vi "Main.vi"() -> ()   [LabVIEW 2016]
uses:
  Composite/Composite Waveform.lvclass
  C:/Users/fflores/Documents/LabVIEW-Open-Projects/Signal Generator OOP/Waveform/Waveform.lvclass
  Sine/Sine.lvclass
  Triangle/Triangle.lvclass
  Waveform/Waveform.lvclass/Waveform.ctl
  Composite/Composite Waveform.lvclass/Composite Waveform.ctl
  Waveform/Waveform.lvclass
panel:
  in  "Refresh Button":bool
  in  "Select Specific Waveform":i32
  in  "Remove Button":bool
  out "Waveform Graph 2":waveform(dbl)(graph)
  in  "Add":bool
  in  "Waveform":enum16{"Sine", "Todas", "Triangle"}(ring)
  in  "stop":bool
  in  "Amplitude":dbl
  in  "Offset":dbl
  in  "Frequency":dbl
  out "Waveform Graph":waveform(dbl)(graph)
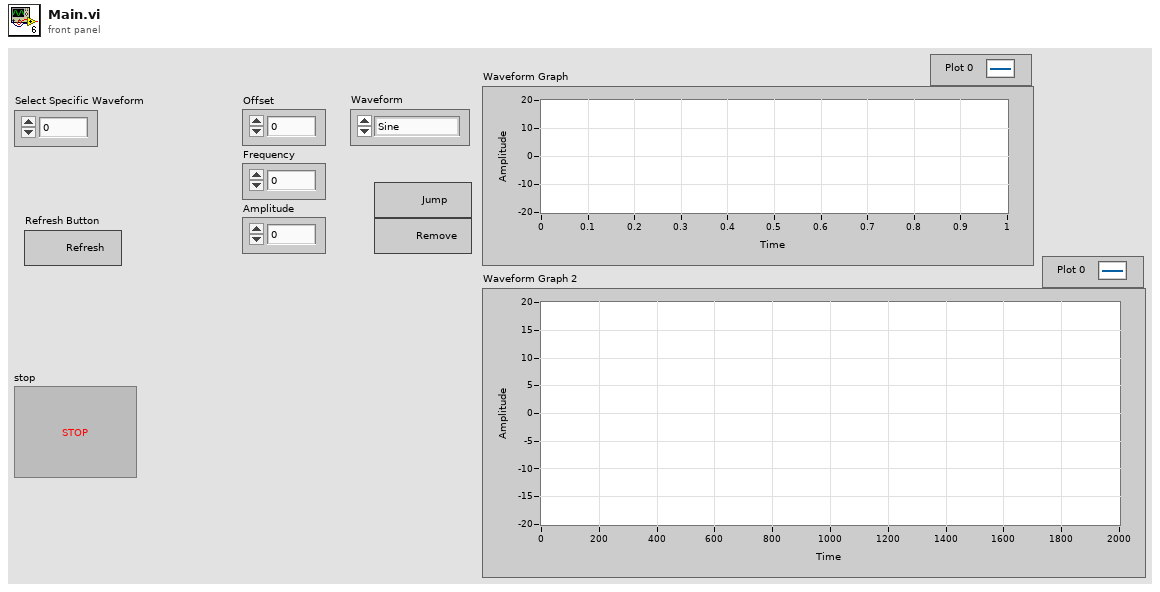
[diagram p1: front panel]
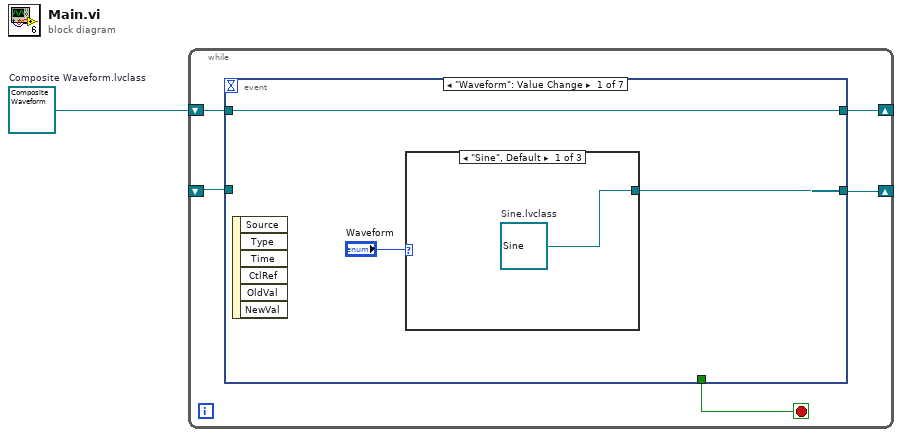
[diagram p0: block diagram]
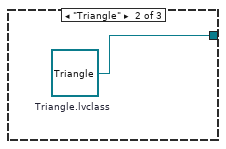
[diagram p2: hidden frame]
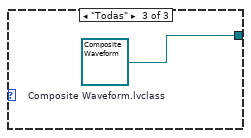
[diagram p3: hidden frame]
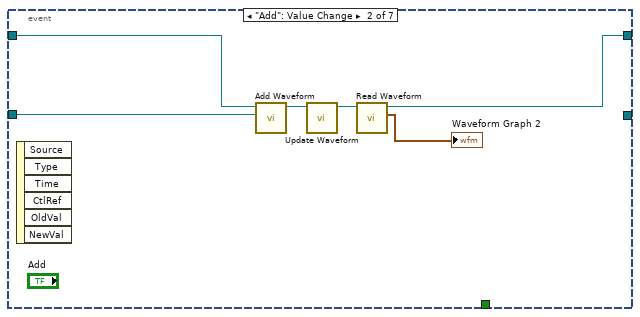
[diagram p4: hidden frame]
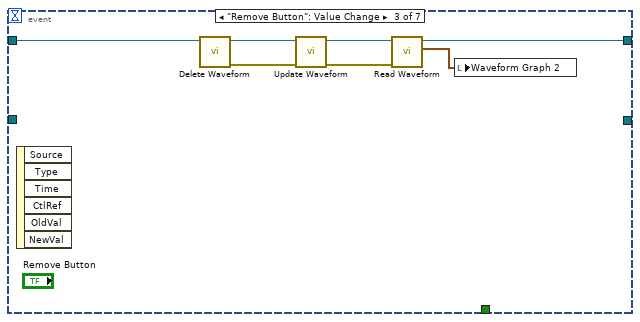
[diagram p5: hidden frame]
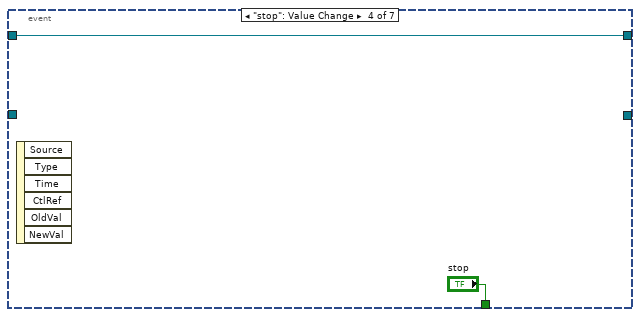
[diagram p6: hidden frame]
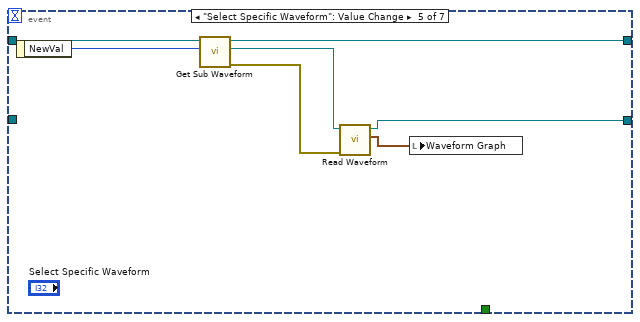
[diagram p7: hidden frame]
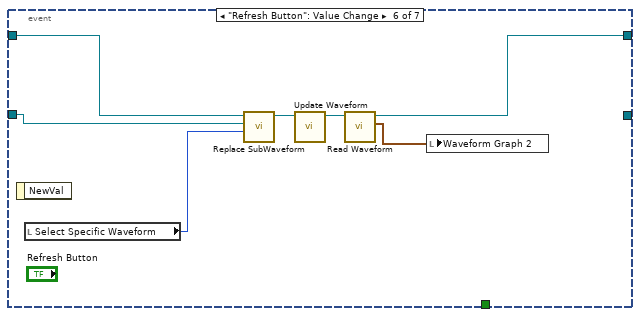
[diagram p8: hidden frame]
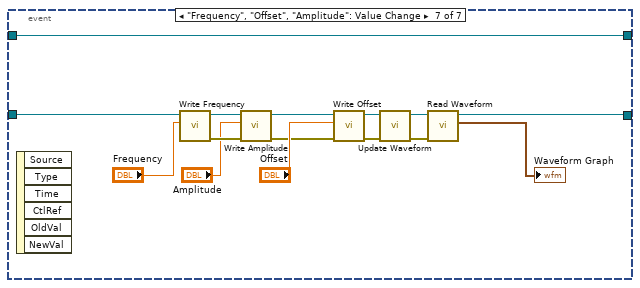
[diagram p9: hidden frame]
diagram:
  w1 = refnum<class "Composite Waveform.lvclass"> refnum  # Composite Waveform.lvclass
  n1 = while {
    shift-right: [w6] -> _
    shift-left: _ -> [w5]
    shift-right: [w3] -> _
    shift-left: w1 -> [w4]
    stop <- w2 stop-if-true
    n2 = event shown="[0] \"Waveform\": Value Change" {
      selector: _ -> [_ _ _ _ _ _ _]
      dyn-events: _ -> [_ _ _ _ _ _ _]
      timeout: _ -> [_ _ _ _ _ _ _]
      tunnel: [w8 _ _ _ w30 _ w43] -> w6
      tunnel: w5 -> [_ w18 _ _ _ w38 w50]
      tunnel: w4 -> [w7 w17 w25 w27 w34 w36 w42]
      tunnel: [w7 w14 w23 w27 w29 w35 w42] -> w3
      tunnel: [_ _ _ "stop" _ _ _] -> w2
      event "Waveform": Value Change {
        n3 = event-data() -> ()  [unwired: 1 in, 6 out]
        n4 = case shown="\"Sine\", Default" "Waveform" {
          tunnel: [w10 w11 w12] -> w8
          frame "Sine", Default {
            w10 = refnum<class "Sine.lvclass"> refnum  # Sine.lvclass
          }
          frame "Triangle" {
            w11 = refnum<class "Triangle.lvclass"> refnum  # Triangle.lvclass
          }
          frame "Todas" {
            w12 = refnum<class "Composite Waveform.lvclass"> refnum  # Composite Waveform.lvclass
          }
        }
      }
      event "Add": Value Change {
        n5 = event-data() -> ()  [unwired: 1 in, 6 out]
        n6 = call "Add Waveform.vi"("Waveform.lvclass"=w18, "Composite Waveform in"=w17) -> ("Composite Waveform out"=w16:refnum<class "Composite Waveform.lvclass">)  [unwired: 8 in, 1 out]
        n7 = call-dynamic "Update Waveform.vi"("Composite Waveform in"=w16) -> ("Composite Waveform out"=w15:refnum<class "Composite Waveform.lvclass">)  [unwired: 9 in, 1 out]
        n8 = call "Read Waveform.vi"("Waveform in"=w15) -> ("Waveform"=→"Waveform Graph 2":waveform(dbl), "Waveform out"=w14:refnum<class "Composite Waveform.lvclass">)  [unwired: 8 in, 1 out]
      }
      event "Remove Button": Value Change {
        n9 = event-data() -> ()  [unwired: 1 in, 6 out]
        n10 = call-dynamic "Delete Waveform.vi"("Composite Waveform in"=w25) -> ("error out"=w20:errorcluster, "Composite Waveform out"=w24:refnum<class "Composite Waveform.lvclass">)  [unwired: 9 in]
        n11 = call-dynamic "Update Waveform.vi"("error in (no error)"=w20, "Composite Waveform in"=w24) -> ("error out"=w19:errorcluster, "Composite Waveform out"=w21:refnum<class "Composite Waveform.lvclass">)  [unwired: 8 in]
        n12 = call "Read Waveform.vi"("error in (no error)"=w19, "Waveform in"=w21) -> ("Waveform"=w22:waveform(dbl), "Waveform out"=w23:refnum<class "Composite Waveform.lvclass">)  [unwired: 7 in, 1 out]
        n13 = local write "Waveform Graph 2"(w22) -> ()
      }
      event "stop": Value Change {
        n14 = event-data() -> ()  [unwired: 1 in, 6 out]
      }
      event "Select Specific Waveform": Value Change {
        n15 = event-data() -> ("NewVal"=w33:i32)  [unwired: 1 in]
        n16 = call "Get Sub Waveform.vi"("index"=w33, "Composite Waveform in"=w34) -> ("error out"=w32:errorcluster, "Waveform.lvclass"=w28:refnum<class "Waveform.lvclass">, "Composite Waveform out"=w29:refnum<class "Composite Waveform.lvclass">)  [unwired: 7 in]
        n17 = call "Read Waveform.vi"("error in (no error)"=w32, "Waveform in"=w28) -> ("Waveform"=w31:waveform(dbl), "Waveform out"=w30:refnum<class "Waveform.lvclass">)  [unwired: 7 in, 1 out]
        n18 = local write "Waveform Graph"(w31) -> ()
      }
      event "Refresh Button": Value Change {
        n19 = event-data() -> ()  [unwired: 1 in, 1 out]
        n20 = local read "Select Specific Waveform"() -> (w39:i32)
        n21 = call "Replace SubWaveform.vi"("Index"=w39, "Waveform.lvclass"=w38, "Composite Waveform in"=w36) -> ("Composite Waveform out"=w41:refnum<class "Composite Waveform.lvclass">)  [unwired: 7 in, 1 out]
        n22 = call-dynamic "Update Waveform.vi"("Composite Waveform in"=w41) -> ("Composite Waveform out"=w40:refnum<class "Composite Waveform.lvclass">)  [unwired: 9 in, 1 out]
        n23 = call "Read Waveform.vi"("Waveform in"=w40) -> ("Waveform"=w37:waveform(dbl), "Waveform out"=w35:refnum<class "Composite Waveform.lvclass">)  [unwired: 8 in, 1 out]
        n24 = local write "Waveform Graph 2"(w37) -> ()
      }
      event "Frequency", "Offset", "Amplitude": Value Change {
        n25 = event-data() -> ()  [unwired: 1 in, 6 out]
        n26 = call "Write Frequency.vi"("Frequency"="Frequency", "Waveform in"=w50) -> ("error out"=w53:errorcluster, "Waveform out"=w52:refnum<class "Waveform.lvclass">)  [unwired: 8 in]
        n27 = call "Write Amplitude.vi"("error in (no error)"=w53, "Amplitude"="Amplitude", "Waveform in"=w52) -> ("error out"=w54:errorcluster, "Waveform out"=w55:refnum<class "Waveform.lvclass">)  [unwired: 7 in]
        n28 = call "Write Offset.vi"("error in (no error)"=w54, "Offset"="Offset", "Waveform in"=w55) -> ("error out"=w44:errorcluster, "Waveform out"=w45:refnum<class "Waveform.lvclass">)  [unwired: 7 in]
        n29 = call-dynamic "Update Waveform.vi"("error in (no error)"=w44, "Waveform in"=w45) -> ("error out"=w47:errorcluster, "Waveform out"=w48:refnum<class "Waveform.lvclass">)  [unwired: 8 in]
        n30 = call "Read Waveform.vi"("error in (no error)"=w47, "Waveform in"=w48) -> ("Waveform"=→"Waveform Graph":waveform(dbl), "Waveform out"=w43:refnum<class "Waveform.lvclass">)  [unwired: 7 in, 1 out]
      }
    }
  }
